vi "Begin.vi"(11 "Image Size":T1=enum."160x120") -> (0 "error out":errorcluster)   [LabVIEW 2012]
doc: "Called before other user functions, this VI is expected to open initial I/O refnums, load in file data, and do all program initialization. Notice that the <B>error out</B> terminal is simply used for data flow. Wiring it to other structures or subVIs ensures that this VI runs first."
uses:
  <vilib>/Rock Robotics/WPI/Camera/WPI_CameraImageSize.ctl
  <vilib>/Rock Robotics/WPI/DriverStation/WPI_DriverStationRobotMode2.ctl
  Robot Global Data.vi
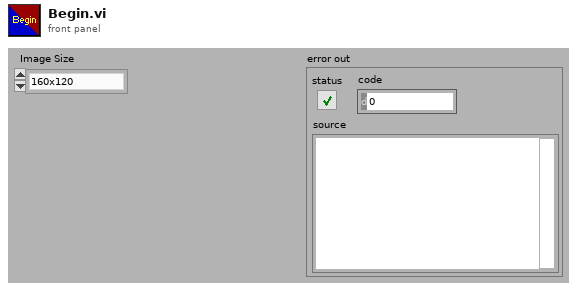
[diagram p1: front panel]
types:
  T1 = typedef "WPI_CameraImageSize.ctl" = enum16{"640x480", "320x240", "160x120"}
  T2 = typedef "WPI_DriverStationRobotMode2.ctl" = enum16{"Autonomous Disabled", "Autonomous Enabled", "Teleop Disabled", "Teleop Enabled", "Timeout", "Finish", "Test Disabled", "Test Enabled"}
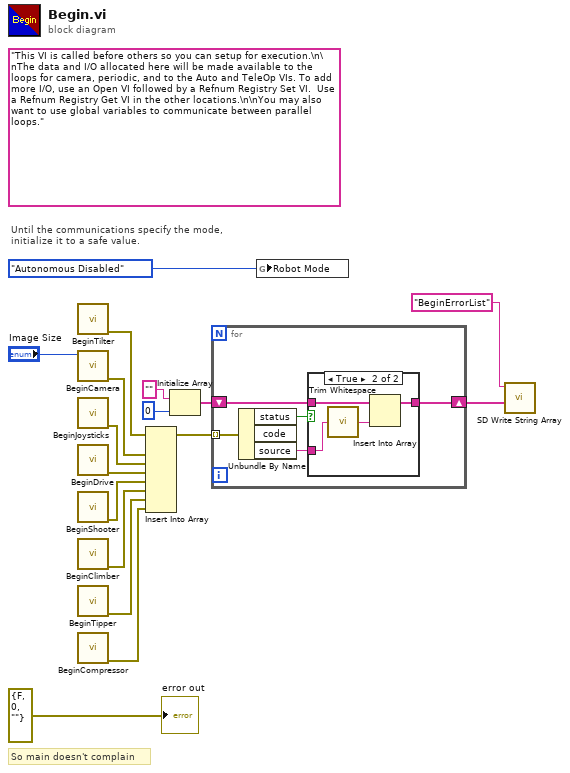
[diagram p0: block diagram]
diagram:
  (unwired) "This VI is called before others so you can setup for execution.\n\nThe data and I/O allocated here will be made available to the loops for camera, periodic, and to the Auto and TeleOp VIs. To add more I/O, use an Open VI followed by a Refnum Registry Set VI.  Use a Refnum Registry Get VI in the other locations.\n\nYou may also want to use global variables to communicate between parallel loops."
  # "So main doesn't complain"
  # "Until the communications specify the mode,\ninitialize it to a safe value."
  n1 = call "BeginTilter.vi"() -> ("Error out array"=w15:errorcluster[])  [unwired: 11 in]
  n2 = call "BeginCamera.vi"("Image Size"="Image Size") -> ("Error Out List"=w14:errorcluster[])  [unwired: 10 in]
  n3 = call "BeginJoysticks.vi"() -> ("Error Out List"=w13:errorcluster[])  [unwired: 11 in]
  n4 = call "BeginDrive.vi"() -> ("Error Out List"=w12:errorcluster[])  [unwired: 11 in]
  n5 = call "BeginShooter.vi"() -> ("Error Out List"=w11:errorcluster[])  [unwired: 11 in]
  n6 = call "BeginClimber.vi"() -> ("Error Out List"=w10:errorcluster[])  [unwired: 11 in]
  n7 = call "BeginTipper.vi"() -> ("Error Out Array"=w9:errorcluster[])  [unwired: 11 in]
  n8 = call "BeginCompressor.vi"() -> ("Error Out Array"=w8:errorcluster[])  [unwired: 11 in]
  n9 = Insert Into Array(array=w15, new element #1=w14, new element #2=w13, new element #3=w12, new element #4=w11, new element #5=w10, new element #6=w9, new element #7=w8) -> (w6:errorcluster[])  [unwired: 1 in]
  n10 = Initialize Array("" ("element"), 0 ("dimension size")) -> (w3:string[])
  n11 = for {
    tunnel: w6 -> [w22] mode=indexing
    shift-right: [w18] -> w1
    shift-left: w3 -> [w19]
    n12 = Unbundle By Name(w22) -> ("status"=w21:bool, "source"=w20:string)  [unwired: 1 out]
    n13 = case shown="True" w21 {
      tunnel: w19 -> [w23 w27]
      tunnel: w20 -> [_ w25]
      tunnel: [w23 w26] -> w18
      frame False {
      }
      frame True {
        n14 = call <vilib>:"Trim Whitespace.vi"("string"=w25) -> ("trimmed string"=w24:string)  [unwired: 1 in]
        n15 = Insert Into Array(array=w27, new element=w24) -> (w26:string[])  [unwired: 1 in]
      }
    }
  }
  n16 = global write "Robot Global Data.vi" "Robot Mode"(WPI_DriverStationRobotMode2."Autonomous Disabled" ("Robot Mode")) -> ()
  n17 = call <vilib>:"SD Write String Array.vi"("String Array"=w1, "Name"="BeginErrorList") -> ()  [unwired: 8 in, 2 out]
  "error out" <- errorcluster {"status"=FALSE, "code"=0, "source"=""} ("error out")
